vi "ADC Start Continue Read.vi"(6 "pGetDataHandle":cluster{}, 7 "FrameSize":i32, 9 "SampleRateHz":i32, 10 "Channel":i8, 11 "DevHandle":i32) -> (3 "function return":i32)   [LabVIEW 2010, in "usb2adc.lvlib"]
doc: "int WINAPI ADC_StartContinueRead(int DevHandle,char Channel,int SampleRateHz,int FrameSize,PADC_GET_DATA_HANDLE pGetDataHandle);"
uses:
  usb2adc.lvlib
  USB2XXX.dll
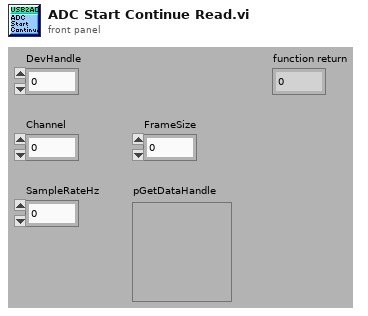
[diagram p1: front panel]
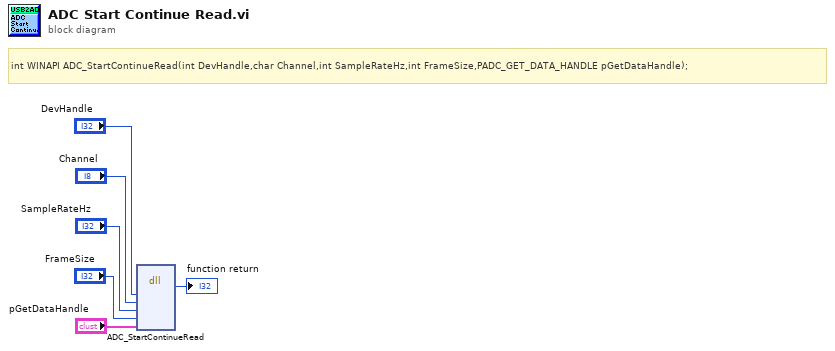
[diagram p0: block diagram]
diagram:
  # "int WINAPI ADC_StartContinueRead(int DevHandle,char Channel,int SampleRateHz,int FrameSize,PADC_GET_DATA_HANDLE pGetDataHandle);"
  n1 = dll-call lib="G:/OtherWork/USB2XXX_Example/trunk/Labview/PublicFiles/usb2adc/USB2XXX.*" fn="ADC_StartContinueRead"("DevHandle"="DevHandle", "Channel"="Channel", "SampleRateHz"="SampleRateHz", "FrameSize"="FrameSize", "pGetDataHandle"="pGetDataHandle") -> (→"function return":i32)  [unwired: 8 in, 2 out]
